vi "示波器2.vi"() -> ()   [LabVIEW 2018]
uses:
  <instrlib>/niScope/Controls/niScope array measurement.ctl
  <instrlib>/niScope/Controls/niScope scalar measurement.ctl
  <instrlib>/niScope/Configure/Trigger/niScope Configure Trigger Edge.vi
  <instrlib>/niScope/Acquire/niScope Multi Read Cluster.vi
  <instrlib>/niScope/Measurements/niScope Fetch Measurement.vi
  <instrlib>/niScope/Measurements/niScope Multi Fetch Array Measurement Cluster.vi
panel:
  out "Waveform From Scope 2":T1(graph) caption="触发通道"
  in  "Channel(s) 2":string="0" caption="触发通道"
  in  "Channel(s)":string="0" caption="采集通道"
  out "Waveform From Scope":T1(graph) caption="采集通道"
  in  "Stop":bool caption="stop"
  in  "Vertical Range (V)":dbl=5.0 format="%_3g"
  in  "Min. Sample Rate":dbl=10000000.0 format="%#_6p"
  in  "Min Record Length":i32=40000
  in  "Vertical Coupling":i32(ring)=1 items=["AC", "DC", "Ground"]
  in  "Trigger Slope":i32(ring) items=["Positive", "Negative"]
  in  "Coupling":u16(ring)=1 items=["AC"=0, "DC"=1, "HF Reject"=3, "LF Reject"=4, "AC Plus HF Reject"=1001]
  in  "Trigger Level (V)":dbl=0.5 caption="Trigger Level" format="%.2f"
  in  "Trigger Modifier":i32(ring)=2 items=["None"=1, "Auto Trigger"=2]
  in  "Input Impedance":u32(ring) items=["1 mega ohm"=0, "50 ohms"=2]
  in  "Tab Control":T2(tab) caption="tab control"
  in  "scalar measurement":T3=4000 caption="Scalar Measurement" items=["None"=4000, "Frequency"=2, "Average Frequency"=1016, "FFT Frequency"=1008, "Period"=3, "Average Period"=1015, "Rise Time"=0, "Fall Time"=1, "Rising Slew Rate"=1010, "Falling Slew Rate"=1011, "Overshoot"=18, "Preshoot"=19, "Voltage RMS"=4, "Voltage Cycle RMS"=16, "AC Estimate"=1012, "FFT Amplitude"=1009, "Voltage Average"=10, "Voltage Cycle Average"=17, "DC Estimate"=1013, "Voltage Max"=6, "Voltage Min"=7, "Voltage Peak-to-Peak"=5, "Voltage High"=8, "Voltage Low"=9, "Voltage Amplitude"=15, "Voltage Top"=1007, "Voltage Base"=1006, "Voltage Base-to-Top"=1017, "Negative Width"=11, "Positive Width"=12, "Negative Duty Cycle"=13, "Positive Duty Cycle"=14, "Integral"=1005, "Area"=1003, "Cycle Area"=1004, "Time Delay"=1014, "Phase Delay"=1018, "Low Ref Volts"=1000, "Mid Ref Volts"=1001, "High Ref Volts"=1002, "Volt. Hist. Mean"=2000, "Volt. Hist. Stdev"=2001, "Volt. Hist. Median"=2003, "Volt. Hist. Mode"=2010, "Volt. Hist. Max"=2005, "Volt. Hist. Min"=2006, "Volt. Hist. Peak-to-Peak"=2002, "Volt. Hist. Mean + Stdev"=2007, "Volt. Hist. Mean + 2 Stdev"=2008, "Volt. Hist. Mean + 3 Stdev"=2009, "Volt. Hist. Hits"=2004, "Volt. Hist. New Hits"=2011, "Time Hist. Mean"=3000, "Time Hist. Stdev"=3001, "Time Hist. Median"=3003, "Time Hist. Mode"=3010, "Time Hist. Max"=3005, "Time Hist. Min"=3006, "Time Hist. Peak-to-Peak"=3002, "Time Hist. Mean + Stdev"=3007, "Time Hist. Mean + 2 Stdev"=3008, "Time Hist. Mean + 3 Stdev"=3009, "Time Hist. Hits"=3004, "Time Hist. New Hits"=3011]
  out "scalar result":dbl caption="Scalar Result"
  in  "Array Measurement":T4=4019 items=["None"=4000, "Last Acq. Histogram"=4001, "Multi Acq. Voltage Histogram"=4004, "Multi Acq. Time Histogram"=4005, "Multi Acq. Average"=4016, "Polynomial Interpolation"=4011, "Array Integral"=4006, "Derivative"=4007, "Inverse"=4008, "Multiply Channels"=4012, "Add Channels"=4013, "Subtract Channels"=4014, "Divide Channels"=4015, "Array Offset"=4025, "Array Gain"=4026, "Hanning Window"=4009, "Flat Top Window"=4010, "Hamming Window"=4020, "Triangle Window"=4023, "Blackman Window"=4024, "FIR Windowed Filter"=4021, "Bessel IIR Filter"=4022, "Butterworth IIR Filter"=4017, "Chebyshev IIR Filter"=4018, "FFT Phase Spectrum"=4002, "FFT Amp. Spectrum (Volts RMS)"=4003, "FFT Amp. Spectrum (dB)"=4019]
  out "array measurement result":T5(graph) caption="Array Measurement Result"
  in  "Resource Name":refnum<k15>="DAQ::1"
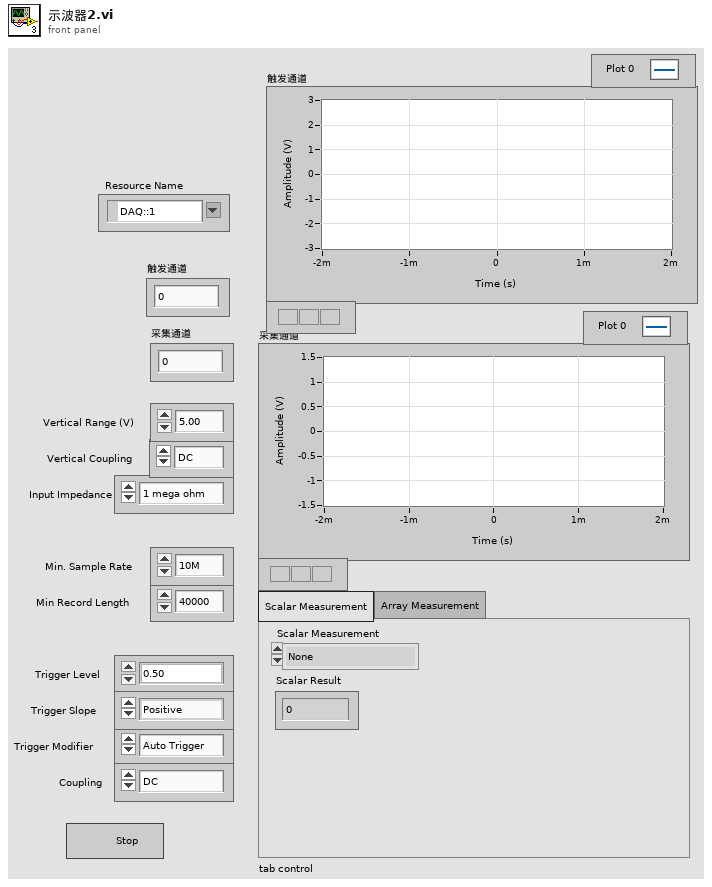
[diagram p1: front panel]
types:
  T1 = cluster{"relativeInitialX":dbl, "xIncrement":dbl, "wfm":dbl[]}[]
  T2 = enum32{"Scalar Measurement", "Array Measurement"}
  T3 = typedef "niScope scalar measurement.ctl" = i32
  T4 = typedef "niScope array measurement.ctl" = i32
  T5 = cluster{"relativeInitialX":dbl, "xIncrement":dbl, "measWfm":dbl[]}[]
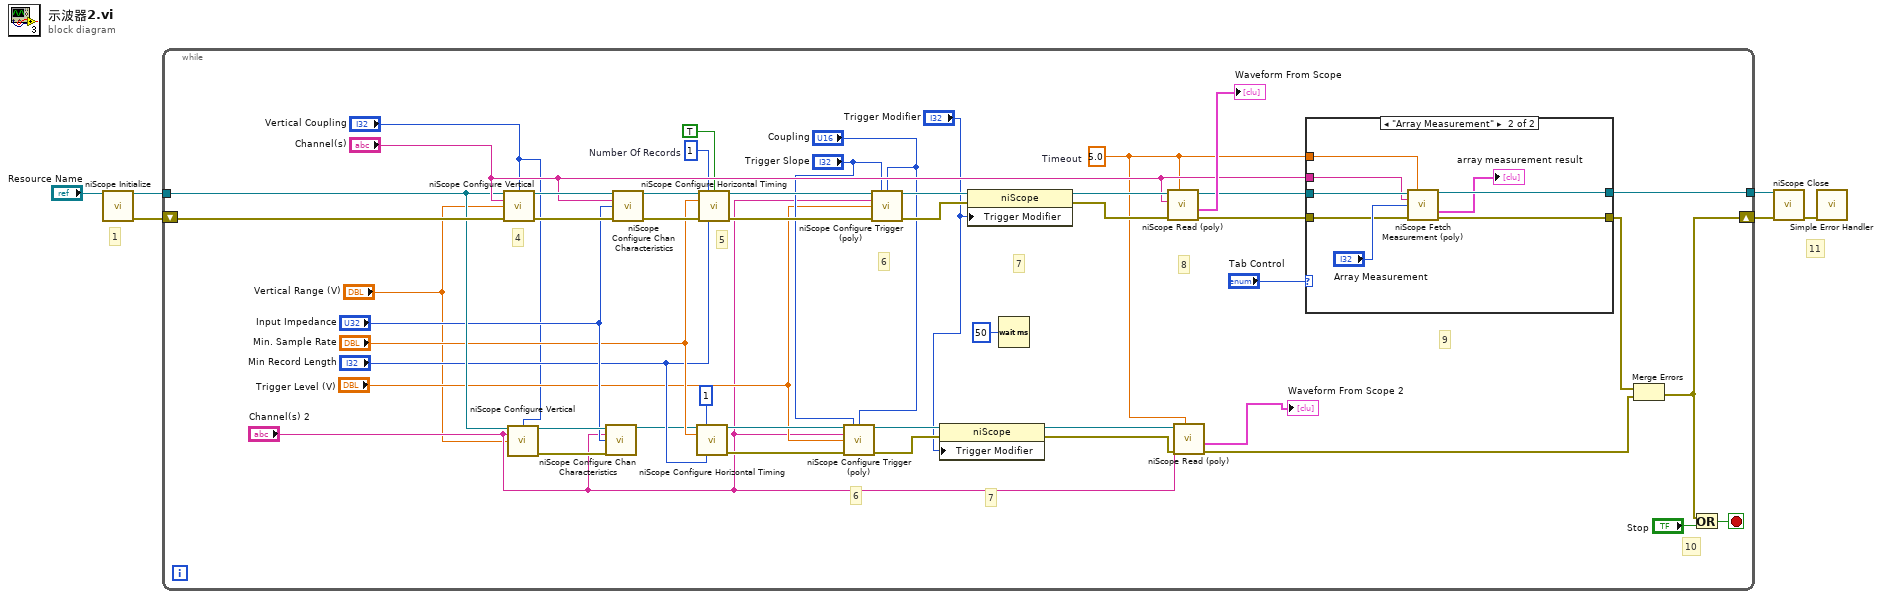
[diagram p0: block diagram]
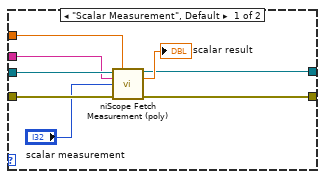
[diagram p2: hidden frame]
diagram:
  # "11"
  # "1"
  n1 = call <instrlib>:"niScope Initialize.vi"("resource name"="Resource Name") -> ("instrument handle"=w4:refnum<k15>, "error out"=w3:errorcluster)  [unwired: 13 in]
  n2 = while {
    tunnel: w4 -> [w32]
    tunnel: [w44] -> w2
    shift-right: [w7] -> w1
    shift-left: w3 -> [w33]
    stop <- w53 stop-if-true
    w36 = 1  # Number Of Records
    w23 = 5.0  # Timeout
    # "6"
    # "7"
    # "9"
    # "8"
    # "6"
    # "5"
    # "4"
    # "10"
    # "7"
    n3 = call <instrlib>:"niScope Configure Vertical.vi"("instrument handle"=w32, "vertical coupling"="Vertical Coupling", "channels"="Channel(s)", "vertical range"="Vertical Range (V)", "error in"=w33) -> ("instrument handle out"=w40:refnum<k15>, "error out"=w41:errorcluster)  [unwired: 9 in]
    n4 = call <instrlib>:"niScope Configure Vertical.vi"("instrument handle"=w32, "vertical coupling"="Vertical Coupling", "channels"="Channel(s) 2", "vertical range"="Vertical Range (V)") -> ("instrument handle out"=w31:refnum<k15>, "error out"=w29:errorcluster)  [unwired: 10 in]
    n5 = call <instrlib>:"niScope Configure Chan Characteristics.vi"("instrument handle"=w31, "channels"="Channel(s) 2", "input impedance"="Input Impedance", "error in"=w29) -> ("instrument handle out"=w24:refnum<k15>)  [unwired: 10 in, 1 out]
    n6 = call <instrlib>:"niScope Configure Chan Characteristics.vi"("instrument handle"=w40, "channels"="Channel(s)", "input impedance"="Input Impedance", "error in"=w41) -> ("instrument handle out"=w38:refnum<k15>, "error out"=w37:errorcluster)  [unwired: 10 in]
    n7 = call <instrlib>:"niScope Configure Horizontal Timing.vi"("instrument handle"=w24, "number of records"=1, "min sample rate"="Min. Sample Rate", "min record length"="Min Record Length") -> ("instrument handle out"=w20:refnum<k15>, "error out"=w16:errorcluster)  [unwired: 10 in]
    n8 = call <instrlib>:"niScope Configure Horizontal Timing.vi"("instrument handle"=w38, "number of records"=w36, "enforce realtime"=TRUE ("Enforce Realtime"), "min sample rate"="Min. Sample Rate", "error in"=w37, "min record length"="Min Record Length") -> ("instrument handle out"=w49:refnum<k15>, "error out"=w50:errorcluster)  [unwired: 8 in]
    n9 = call-poly <instrlib>:"niScope Configure Trigger (poly).vi"("instrument handle"=w20, "trigger slope"="Trigger Slope", "trigger coupling"="Coupling", "trigger source"="Channel(s) 2", "trigger level"="Trigger Level (V)", "error in"=w16) -> ("instrument handle out"=w22:refnum<k15>, "error out"=w21:errorcluster)  [unwired: 8 in]
    n10 = call-poly <instrlib>:"niScope Configure Trigger (poly).vi"("instrument handle"=w49, "trigger slope"="Trigger Slope", "trigger coupling"="Coupling", "trigger source"="Channel(s) 2", "trigger level"="Trigger Level (V)", "error in"=w50) -> ("instrument handle out"=w46:refnum<k15>, "error out"=w45:errorcluster)  [unwired: 8 in]
    n11 = property class="niScope"(reference=w22, error in=w21, "Trigger Modifier"="Trigger Modifier") -> (reference out=w14:refnum<k15>, error out=w12:errorcluster)
    n12 = property class="niScope"(reference=w46, error in=w45, "Trigger Modifier"="Trigger Modifier") -> (reference out=w42:refnum<k15>, error out=w43:errorcluster)
    n13 = Wait (ms)(milliseconds to wait=u32 50 ("Millisecond Multiple")) -> ()  [unwired: 1 out]
    n14 = call-poly <instrlib>:"niScope Read (poly).vi"("timeout"=w23, "error in"=w43, "channels"="Channel(s)", "instrument handle"=w42) -> ("error out"=w47:errorcluster, "waveform"=→"Waveform From Scope":T1, "instrument handle out"=w48:refnum<k15>)  [unwired: 4 in, 1 out]
    n15 = call-poly <instrlib>:"niScope Read (poly).vi"("timeout"=w23, "error in"=w12, "channels"="Channel(s) 2", "instrument handle"=w14) -> ("error out"=w8:errorcluster, "waveform"=→"Waveform From Scope 2":T1)  [unwired: 4 in, 2 out]
    n16 = case shown="\"Array Measurement\"" "Tab Control" {
      tunnel: [w61 w70] -> w44
      tunnel: [w60 w68] -> w9
      tunnel: w48 -> [w59 w66]
      tunnel: w47 -> [w58 w65]
      tunnel: "Channel(s)" -> [w56 w64]
      tunnel: w23 -> [w55 w63]
      frame "Scalar Measurement", Default {
        n17 = call-poly <instrlib>:"niScope Fetch Measurement (poly).vi"("instrument handle"=w59, "timeout"=w55, "channels"=w56, "scalar measurement"="scalar measurement", "error in"=w58) -> ("instrument handle out"=w61:refnum<k15>, "result"=→"scalar result":dbl, "error out"=w60:errorcluster)  [unwired: 8 in]
      }
      frame "Array Measurement" {
        n18 = call-poly <instrlib>:"niScope Fetch Measurement (poly).vi"("instrument handle"=w66, "timeout"=w63, "channels"=w64, "array measurement"="Array Measurement", "error in"=w65) -> ("instrument handle out"=w70:refnum<k15>, "meas waveform"=→"array measurement result":T5, "error out"=w68:errorcluster)  [unwired: 7 in, 1 out]
      }
    }
    n19 = Merge Errors(w9, w8) -> (w7:errorcluster)
    n20 = Or(x=w7, y="Stop") -> (x .or. y?=w53:bool)
  }
  n21 = call <instrlib>:"niScope Close.vi"("instrument handle"=w2, "error in"=w1) -> ("error out"=w5:errorcluster)  [unwired: 13 in]
  n22 = call <vilib>:"Simple Error Handler.vi"("error in (no error)"=w5) -> ()  [unwired: 4 in, 5 out]
